vi "Create Container.vi"(8 "Error In":errorcluster, 11 "Tab Widget Builder in":refnum<class "Tab Widget Builder.lvclass">) -> (0 "Error Out":errorcluster, 2 "Container":refnum<class "QWidget.lvclass">, 3 "Tab Widget Builder out":refnum<class "Tab Widget Builder.lvclass">)   [LabVIEW 2014, in "Tab Widget Builder.lvclass"]
doc: "Implements the interface provided by Abstract Widget Builder.\n\n\nCopyright (c) 2019 Sze Howe Koh.\nThis code is licensed under the MIT license."
uses:
  Tab Widget Builder.lvclass
  <vilib>/addons/LQ/Qt Widgets/QWidget/QWidget.lvclass
  <vilib>/addons/LQ/Qt Widgets/QTabWidget/QTabWidget.lvclass
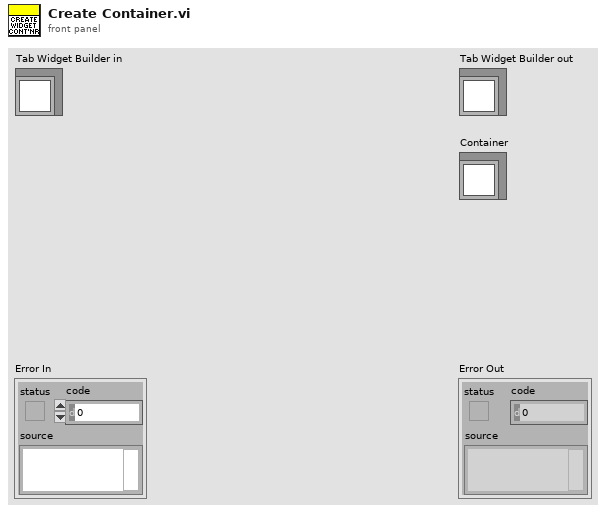
[diagram p1: front panel]
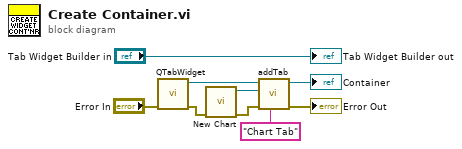
[diagram p0: block diagram]
diagram:
  n1 = call <vilib>:"QTabWidget.vi"("Error In"="Error In") -> ("Error Out"=w3:errorcluster, "New QTabWidget"=w5:refnum<class "QTabWidget.lvclass">)  [unwired: 9 in]
  n2 = call "New Chart.vi"("Error In"=w3) -> ("Error Out"=w2:errorcluster, "New LQChart"=w6:refnum<class "LQChart.lvclass">)  [unwired: 9 in]
  n3 = call <vilib>:"addTab.vi"("label"="Chart Tab", "Error In"=w2, "widget"=w6, "QTabWidget In"=w5) -> ("Error Out"=→"Error Out":errorcluster, "QTabWidget Out"=→"Container":refnum<class "QTabWidget.lvclass">)  [unwired: 5 in, 1 out]
  "Tab Widget Builder out" <- "Tab Widget Builder in"
